vi "Apply Frequency Weighting.vi"(0 "spectrum":dbl[](array[numeric]) format="%.2f", 1 "df [Hz]":dbl format="%.2f", 2 "weighting filter":u16(ring) items=["Linear", "A-weighting", "B-weighting", "C-weighting"], 3 "dB On (T)":bool=TRUE, 4 "spectrum type":enum16{"Power", "Amplitude"}(ring)) -> (5 "frequency weighted spectrum":dbl[](array[numeric]) format="%.2f")   [LabVIEW 2017]
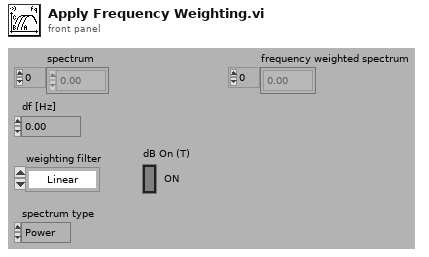
[diagram p1: front panel]
types:
  T1 = typedef "svc_Weighting Filter Text Ring.ctl" = u16
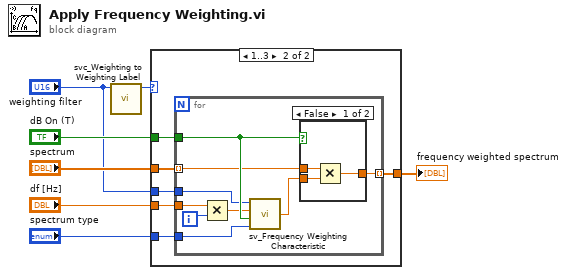
[diagram p0: block diagram]
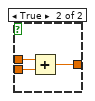
[diagram p3: hidden frame]
diagram:
  n1 = call <vilib>:"svc_Weighting to Weighting Label.vi"("weighting filter"="weighting filter") -> ("weighting enum"=w2:T1)  [unwired: 9 in, 1 out]
  n2 = case shown="1..3" w2 {
    tunnel: "spectrum" -> [w8 w14]
    tunnel: "dB On (T)" -> [_ w13]
    tunnel: [w8 w12] -> w7
    tunnel: "df [Hz]" -> [_ w11]
    tunnel: "spectrum type" -> [_ w10]
    tunnel: "weighting filter" -> [_ w9]
    frame 0, Default {
    }
    frame 1..3 {
      n3 = for {
        tunnel: w11 -> [w23]
        tunnel: w14 -> [w20] mode=indexing
        tunnel: w13 -> [w21]
        tunnel: [w18] -> w12 mode=indexing
        tunnel: w10 -> [w15]
        tunnel: w9 -> [w16]
        i -> [w22]
        n4 = Multiply(x=w23, y=w22) -> (x*y=w17:dbl)
        n5 = call <vilib>:"sv_Frequency Weighting Characteristic.vi"("spectrum type"=w15, "dB On (T)"=w21, "frequency [Hz]"=w17, "weighting filter"=w16) -> ("relative response level"=w19:dbl)
        n6 = case shown="False" w21 {
          tunnel: w20 -> [w26 w29]
          tunnel: w19 -> [w25 w28]
          tunnel: [w24 w27] -> w18
          frame False {
            n7 = Multiply(x=w26, y=w25) -> (x*y=w24:dbl)
          }
          frame True {
            n8 = Add(x=w29, y=w28) -> (x+y=w27:dbl)
          }
        }
      }
    }
  }
  "frequency weighted spectrum" <- w7
